vi "file_waring_m.vi"(2 "item not found":string, 4 "index":i16) -> ()   [LabVIEW 2010]
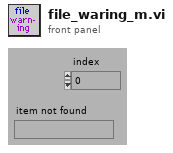
[diagram p1: front panel]
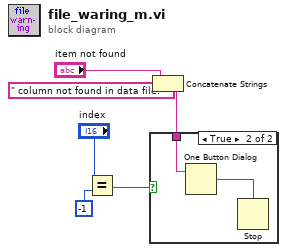
[diagram p0: block diagram]
diagram:
  n1 = Equal?(x="index", y=-1) -> (x = y?=w4:bool)
  n2 = Concatenate Strings("item not found", " column not found in data file.") -> (w1:string)
  n3 = case shown="True" w4 {
    tunnel: w1 -> [_ w7]
    frame False {
    }
    frame True {
      n4 = One Button Dialog(message=w7) -> (true=w8:bool)  [unwired: 1 in]
      n5 = Stop(stop? (T)=w8) -> ()
    }
  }
